vi "外部交互全局变量.vi"() -> ()   [LabVIEW 2022 SP3, in "环境动力监测库.lvlib"]
uses:
  <vilib>/Plasmionique/MB Master/MB_Master/MB_Master.lvclass
panel:
  in  "告警交互":T1
  out "初始化":bool
  out "动力环境":T2
  in  "权限等级":enum16{"一级权限", "二级权限", "三级权限", "超级权限"}(ring)
  in  "与V采配水PLC交互全局":T4={"状态"={"R0"=0, "R1"=0, "R2"=0, "R3"=0, "R4"=0, "R5"=0, "R6"=0, "R7"=0, "R8"=0, "R9"=0, "R10"=0, "R11"=0, "R12"=0, "R13"=0, "R14"=0, "R15"=0, "R16"=0, "R17"=0, "R18"=0, "R19"=0, "R20"=0, "R21"=0, "R22"=0, "R23"=0, "R24"=0, "R25"=0, "R26"=0, "R27"=0, "R28"=0, "R29"=0, "R30"=0, "R31"=0, "R32"=0, "R33"=0, "R34"=0, "R35"=0, "R36"=0, "R37"=0, "R38"=0, "R39"=0, "R40"=0, "R41"=0, "R42"=0, "R43"=0, "R44"=0, "R45"=0, "R46"=0, "R47"=0, "R48"=0, "R49"=0, "R50"=0, "R51"=0, "R52"=0, "R53"=0, "R54"=0, "R55"=0, "R56"=0, "R57"=0, "R58"=0, "R59"=0, "R60"=0, "R61"=0, "R62"=0, "R63"=0, "R64"=0, "R65"=0, "R66"=0, "R67"=0, "R68"=0, "R69"=0}, "输入状态"=[], "输出状态"=[], "报警簇"=[], "参数设置"={"R100"=0, "R101"=0, "R102"=0, "R103"=0, "R104"=0, "R105"=0, "R106"=0, "R107"=0, "R108"=0, "R109"=0, "R110"=0, "R111"=0, "R112"=0, "R113"=0, "R114"=0, "R115"=0, "R116"=0, "R117"=0, "R118"=0, "R119"=0, "R120"=0, "R121"=0, "R122"=0, "R123"=0, "R124"=0}, "转换值"={"AD0"=0.0, "AD1"=0.0, "AD2"=0.0, "AD3"=0.0, "AD4"=0.0, "AD5"=0.0}, "看门狗启用"=FALSE, "氨氮模块名称"="", "总磷模块名称"="", "采配水模块类型"=enum."V4"}
  in  "与ZLAN交互全局":T5 {"环境变量"."湿度" format="%.0f %%RH"; "环境变量"."室温" format="%.2f ℃"; "环境变量"."蓄电池电压" format="%.2f V"}
  in  "与G采配水PLC交互全局":T6
  in  "与系统交互":T7
  in  "应用环境":enum16{"固定站", "微站", "浮标", "浮船"}(ring)
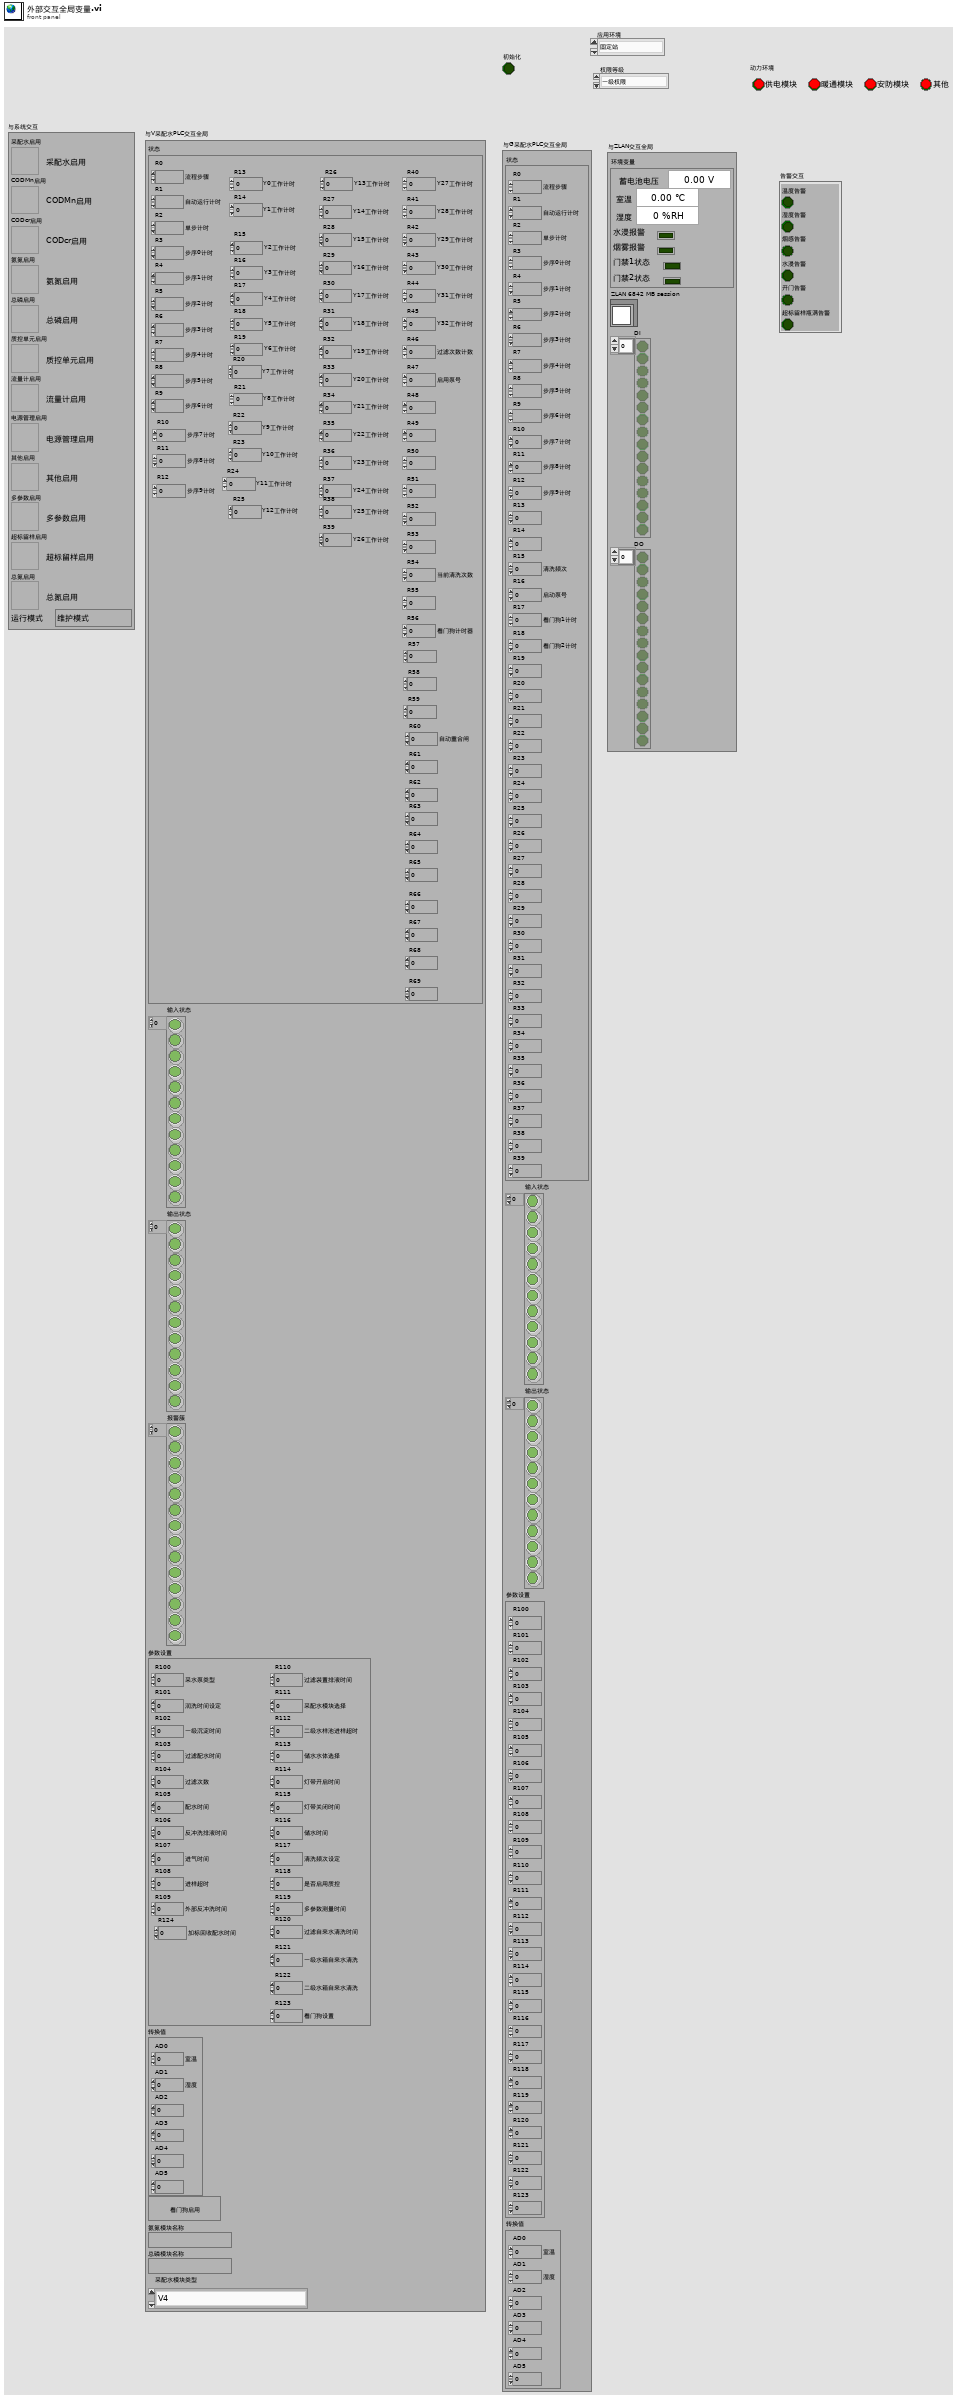
[diagram p1: front panel]
types:
  T1 = cluster{"温度告警":bool, "湿度告警":bool, "烟感告警":bool, "水浸告警":bool, "开门告警":bool, "超标留样瓶满告警":bool}
  T2 = cluster{"供电模块":bool, "暖通模块":bool, "安防模块":bool, "其他":bool}
  T3 = typedef "采配水类型.ctl" = enum16{"V1", "V2", "V3", "V4", "室内V1", "室内V2", "固定站V1", "固定站V2", "浮船V1", "浮船V2", "养殖尾水", "广东华南所"}
  T4 = cluster{"状态":cluster{"R0":i16, "R1":i16, "R2":i16, "R3":i16, "R4":i16, "R5":i16, "R6":i16, "R7":i16, "R8":i16, "R9":i16, "R10":i16, "R11":i16, "R12":i16, "R13":i16, "R14":i16, "R15":i16, "R16":i16, "R17":i16, "R18":i16, "R19":i16, "R20":i16, "R21":i16, "R22":i16, "R23":i16, "R24":i16, "R25":i16, "R26":i16, "R27":i16, "R28":i16, "R29":i16, "R30":i16, "R31":i16, "R32":i16, "R33":i16, "R34":i16, "R35":i16, "R36":i16, "R37":i16, "R38":i16, "R39":i16, "R40":i16, "R41":i16, "R42":i16, "R43":i16, "R44":i16, "R45":i16, "R46":i16, "R47":i16, "R48":i16, "R49":i16, "R50":i16, "R51":i16, "R52":i16, "R53":i16, "R54":i16, "R55":i16, "R56":i16, "R57":i16, "R58":i16, "R59":i16, "R60":i16, "R61":i16, "R62":i16, "R63":i16, "R64":i16, "R65":i16, "R66":i16, "R67":i16, "R68":i16, "R69":i16}, "输入状态":bool[], "输出状态":bool[], "报警簇":bool[], "参数设置":cluster{"R100":i16, "R101":i16, "R102":i16, "R103":i16, "R104":i16, "R105":i16, "R106":i16, "R107":i16, "R108":i16, "R109":i16, "R110":i16, "R111":i16, "R112":i16, "R113":i16, "R114":i16, "R115":i16, "R116":i16, "R117":i16, "R118":i16, "R119":i16, "R120":i16, "R121":i16, "R122":i16, "R123":i16, "R124":i16}, "转换值":cluster{"AD0":sgl, "AD1":sgl, "AD2":sgl, "AD3":sgl, "AD4":sgl, "AD5":sgl}, "看门狗启用":bool, "氨氮模块名称":string, "总磷模块名称":string, "采配水模块类型":T3}
  T5 = cluster{"环境变量":cluster{"蓄电池电压":dbl, "室温":dbl, "湿度":dbl, "水浸报警":bool, "烟雾报警":bool, "门禁1状态":bool, "门禁2状态":bool}, "ZLAN 6842 MB session":refnum<class "MB_Master.lvclass">, "DI":bool[], "DO":bool[]}
  T6 = cluster{"状态":cluster{"R0":i16, "R1":i16, "R2":i16, "R3":i16, "R4":i16, "R5":i16, "R6":i16, "R7":i16, "R8":i16, "R9":i16, "R10":i16, "R11":i16, "R12":i16, "R13":i16, "R14":i16, "R15":i16, "R16":i16, "R17":i16, "R18":i16, "R19":i16, "R20":i16, "R21":i16, "R22":i16, "R23":i16, "R24":i16, "R25":i16, "R26":i16, "R27":i16, "R28":i16, "R29":i16, "R30":i16, "R31":i16, "R32":i16, "R33":i16, "R34":i16, "R35":i16, "R36":i16, "R37":i16, "R38":i16, "R39":i16}, "输入状态":bool[], "输出状态":bool[], "参数设置":cluster{"R100":i16, "R101":i16, "R102":i16, "R103":i16, "R104":i16, "R105":i16, "R106":i16, "R107":i16, "R108":i16, "R109":i16, "R110":i16, "R111":i16, "R112":i16, "R113":i16, "R114":i16, "R115":i16, "R116":i16, "R117":i16, "R118":i16, "R119":i16, "R120":i16, "R121":i16, "R122":i16, "R123":i16}, "转换值":cluster{"AD0":sgl, "AD1":sgl, "AD2":sgl, "AD3":sgl, "AD4":sgl, "AD5":sgl}}
  T7 = cluster{"采配水启用":bool, "CODMn启用":bool, "CODcr启用":bool, "氨氮启用":bool, "总磷启用":bool, "质控单元启用":bool, "流量计启用":bool, "电源管理启用":bool, "其他启用":bool, "多参数启用":bool, "超标留样启用":bool, "总氮启用":bool, "运行模式":enum16{"维护模式", "常规模式", "应急模式", "质控模式"}}
diagram:
